vi "Write Samples.vi"(8 "error in (no error)":errorcluster, 10 "Samples":dbl, 11 "Stimulus in":refnum<class "Stimulus.lvclass">) -> (0 "error out":errorcluster, 3 "Stimulus out":refnum<class "Stimulus.lvclass">)   [LabVIEW 2015, in "Stimulus.lvclass"]
uses:
  Stimulus.lvclass
  Stimulus.lvclass/Stimulus.ctl
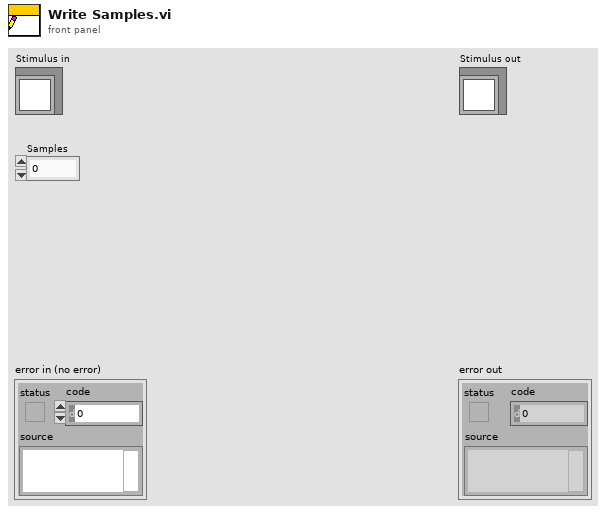
[diagram p1: front panel]
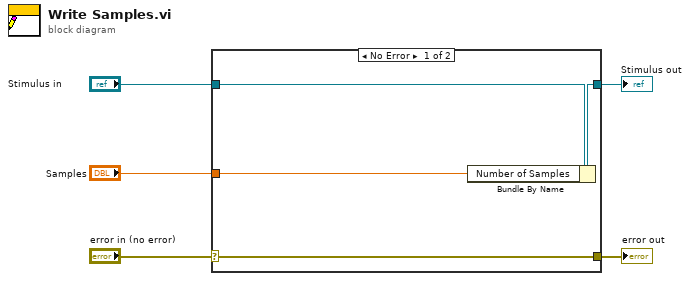
[diagram p0: block diagram]
diagram:
  n1 = case shown="No Error" "error in (no error)" {
    selector: "error in (no error)" -> [w9 w10]
    tunnel: [w9 w10] -> w4
    tunnel: [w7 w11] -> w2
    tunnel: "Stimulus in" -> [w8 w11]
    tunnel: "Samples" -> [w6 _]
    frame No Error {
      n2 = Bundle By Name(cluster=w8, "Number of Samples"=w6) -> (w7:refnum<class "Stimulus.lvclass">)
    }
    frame Error {
    }
  }
  "error out" <- w4
  "Stimulus out" <- w2
